vi "Get Module Config.vi"(8 "error in (no error)":errorcluster, 11 "9237 in":refnum<class "9237.lvclass">) -> (0 "error out":errorcluster, 2 "Config Channels":dbl[](array[numeric]), 3 "9237 out":refnum<class "9237.lvclass">)   [LabVIEW 2017, in "Modules.lvlib" / "9237.lvclass"]
uses:
  9237.lvclass
  9237.lvclass/9237.ctl
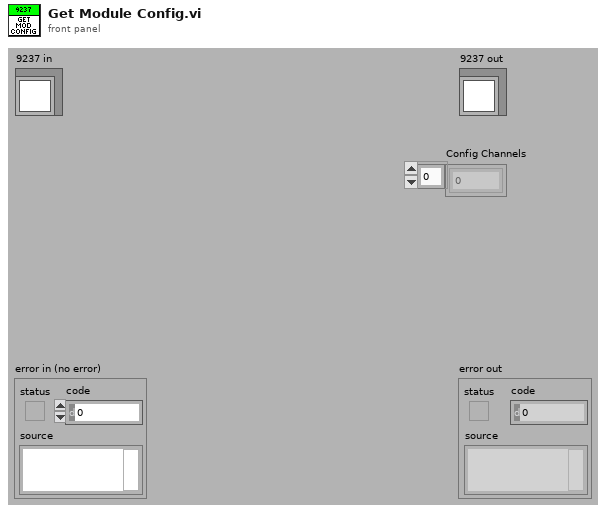
[diagram p1: front panel]
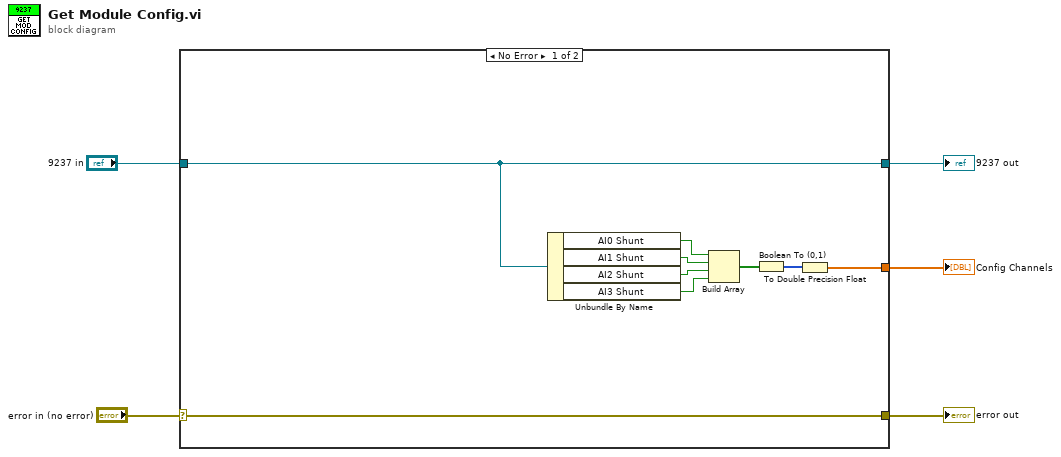
[diagram p0: block diagram]
diagram:
  n1 = case shown="No Error" "error in (no error)" {
    selector: "error in (no error)" -> [w14 w16]
    tunnel: "9237 in" -> [w13 w15]
    tunnel: [w14 w16] -> w3
    tunnel: [w13 w15] -> w2
    tunnel: [w6 _] -> w1
    frame No Error {
      n2 = Unbundle By Name(w13) -> ("AI0 Shunt"=w12:bool, "AI1 Shunt"=w11:bool, "AI2 Shunt"=w10:bool, "AI3 Shunt"=w9:bool)
      n3 = Build Array(w12, w11, w10, w9) -> (w8:bool[])
      n4 = Boolean To (0,1)(Boolean=w8) -> (0, 1=w7:i16[])
      n5 = To Double Precision Float(number=w7) -> (double precision float=w6:dbl[])
    }
    frame Error {
    }
  }
  "error out" <- w3
  "9237 out" <- w2
  "Config Channels" <- w1
